vi "conf2gui.vi"(1 "bad conf":sgl[](array[numeric]), 2 "good conf":sgl[](array[numeric])) -> (0 "ui info":T1)   [LabVIEW 2024]
uses:
  <vilib>/Analysis/NI_AALBase.lvlib
  <vilib>/Analysis/baseanly.llb/Mean (DBL).vi
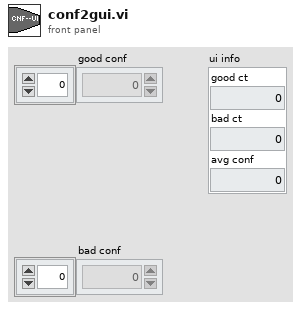
[diagram p1: front panel]
types:
  T1 = cluster{"good ct":i32, "bad ct":i32, "avg conf":dbl}
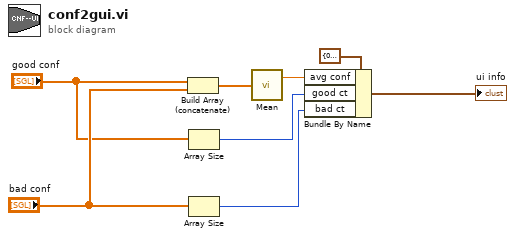
[diagram p0: block diagram]
diagram:
  n1 = Build Array (concatenate)("good conf", "bad conf") -> (w1:sgl[])
  n2 = Array Size(array="good conf") -> (size(s)=w6:i32)
  n3 = Array Size(array="bad conf") -> (size(s)=w7:i32)
  n4 = call-poly <vilib>:"Mean.vi"("X"=w1) -> ("mean"=w5:dbl)  [unwired: 1 out]
  n5 = Bundle By Name(cluster=T1 {"good ct"=0, "bad ct"=0, "avg conf"=0.0}, "avg conf"=w5, "good ct"=w6, "bad ct"=w7) -> (→"ui info":T1)
